vi "Scan_Frequency_Range_NEW.vi"() -> ()   [LabVIEW 2010]
uses:
  <vilib>/Utility/file.llb/Write To Spreadsheet File (DBL).vi
panel:
  out "Error Phase Shift":cluster{dbl[], dbl[]}(graph)
  out "Error Amplitude":cluster{dbl[], dbl[]}(graph)
  out "Phase Shift":cluster{dbl[], dbl[]}(graph)
  out "Amplitude":cluster{dbl[], dbl[]}(graph)
  in  "Path":path
  in  "Wait [s]":dbl
  in  "Stepsize[Hz]":dbl
  in  "Stop Frequency[Hz]":dbl
  in  "Start Frequency [Hz]":dbl
  out "error out":errorcluster
  in  "error in (no error)":errorcluster
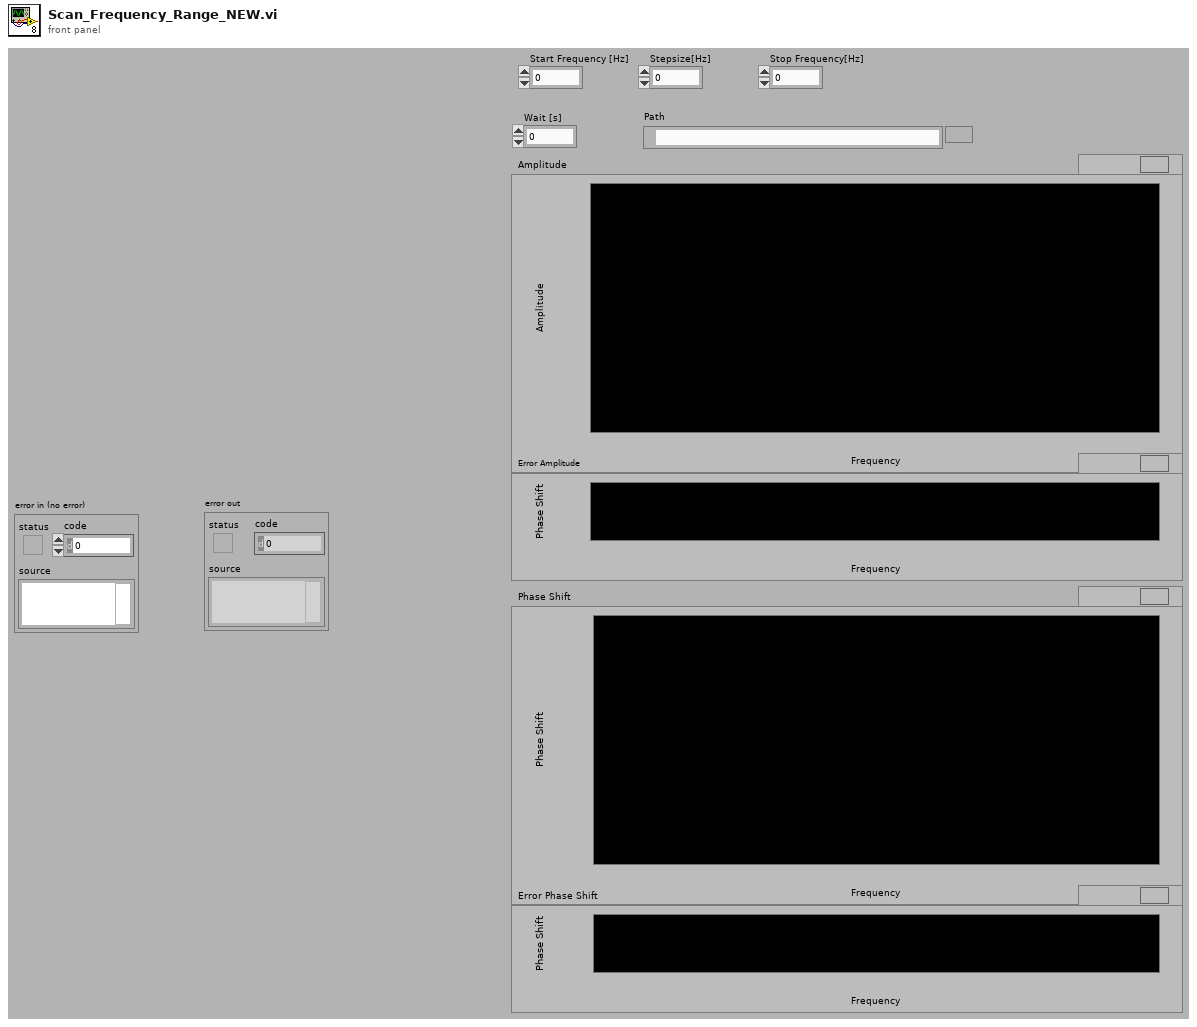
[diagram p1: front panel]
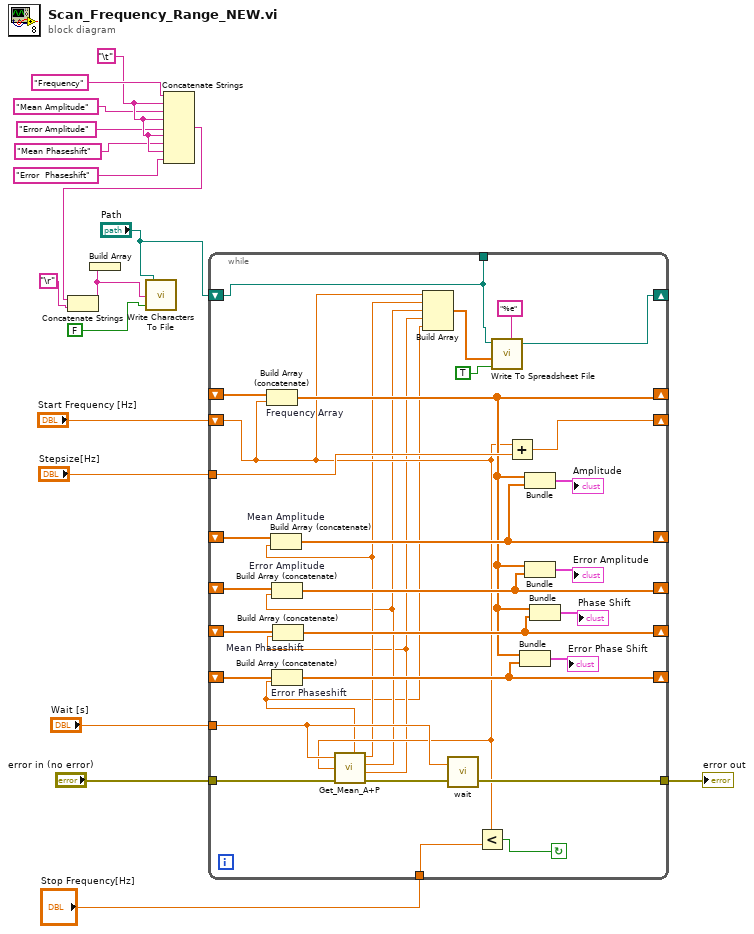
[diagram p0: block diagram]
diagram:
  w7 = "\t"
  n1 = Concatenate Strings("Frequency", w7, "Mean Amplitude", w7, "Error Amplitude", w7, "Mean Phaseshift", w7, "Error  Phaseshift") -> (w2:string)
  n2 = Concatenate Strings(w2, "\r") -> (w9:string)
  n3 = Build Array(w9) -> ()  [unwired: 1 out]
  n4 = call <vilib>:"Write Characters To File.vi"("append to file? (new file:F)"=FALSE, "character string"=w9, "file path (dialog if empty)"="Path") -> ()  [unwired: 2 in, 1 out]
  n5 = while {
    tunnel: "error in (no error)" -> [w49]
    tunnel: [w47] -> w16
    tunnel: "Wait [s]" -> [w39]
    shift-right: [w46] -> _
    shift-left: "Start Frequency [Hz]" -> [w25]
    tunnel: "Stepsize[Hz]" -> [w45]
    tunnel: "Stop Frequency[Hz]" -> [w44]
    tunnel: [w18] -> _
    shift-right: [w27] -> _
    shift-left: _ -> [w40]
    shift-right: [w33] -> _
    shift-left: _ -> [w38]
    shift-right: [w29] -> _
    shift-left: _ -> [w37]
    shift-right: [w31] -> _
    shift-left: _ -> [w36]
    shift-right: [w26] -> _
    shift-left: _ -> [w35]
    shift-right: [w19] -> _
    shift-left: "Path" -> [w18]
    stop <- w43 continue-if-true
    n6 = Build Array (concatenate) "Frequency Array"(w40, w25) -> (w27:dbl[])
    n7 = call "Get_Mean_A+P.vi"("Wait"=w39, "Frequency"=w25, "error in (no error)"=w49) -> ("Mean Amplitude"=w24:dbl, "Error Amplitude"=w23:dbl, "Mean Phase Shift"=w22:dbl, "error out"=w48:errorcluster, "Error Phase Shift"=w21:dbl)
    n8 = Build Array (concatenate) "Mean Amplitude"(w38, w24) -> (w33:dbl[])
    n9 = Build Array (concatenate) "Error Amplitude"(w37, w23) -> (w29:dbl[])
    n10 = Build Array (concatenate) "Error Phaseshift"(w35, w21) -> (w26:dbl[])
    n11 = Build Array (concatenate) "Mean Phaseshift"(w36, w22) -> (w31:dbl[])
    n12 = Build Array(w25, w24, w23, w22, w21) -> (w20:dbl[])
    n13 = call "wait.vi"("error in"=w48, "Wartezeit in Sek"=w39) -> ("error out"=w47:errorcluster)  [unwired: 1 in]
    n14 = Less?(x=w25, y=w44) -> (x < y?=w43:bool)
    n15 = call-poly <vilib>:"Write To Spreadsheet File.vi"("format (%.3f)"="%e", "append to file? (new file:F)"=TRUE, "1D data"=w20, "file path (dialog if empty)"=w18) -> ("new file path (Not A Path if cancelled)"=w19:path)  [unwired: 4 in]
    n16 = Add(x=w25, y=w45) -> (x+y=w46:dbl)
    n17 = Bundle(w27, w26) -> (→"Error Phase Shift":cluster{dbl[], dbl[]})  [unwired: 1 in]
    n18 = Bundle(w27, w33) -> (→"Amplitude":cluster{dbl[], dbl[]})  [unwired: 1 in]
    n19 = Bundle(w27, w29) -> (→"Error Amplitude":cluster{dbl[], dbl[]})  [unwired: 1 in]
    n20 = Bundle(w27, w31) -> (→"Phase Shift":cluster{dbl[], dbl[]})  [unwired: 1 in]
  }
  "error out" <- w16
